vi "Background Color Read.vi"(8 "error in (no error)":errorcluster, 11 "3D Plot.lvclass in":refnum<class "3D Plot.lvclass">) -> (0 "error out":errorcluster, 1 "Plot Area Color":u32(colorbox), 3 "3D Plot.lvclass out":refnum<class "3D Plot.lvclass">)   [LabVIEW 2020, in "3D Plot.lvclass"]
uses:
  <vilib>/Math Plots/3D Math Plots/3D Plot/3D Plot/3D Plot.lvclass
  <vilib>/Math Plots/3D Math Plots/3D Plot/3D Plot/3D Plot.lvclass/3D Plot.ctl
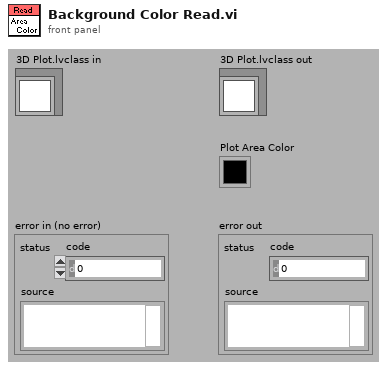
[diagram p1: front panel]
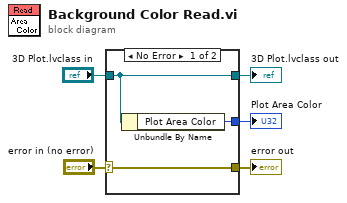
[diagram p0: block diagram]
diagram:
  n1 = case shown="No Error" "error in (no error)" {
    selector: "error in (no error)" -> [w7 w9]
    tunnel: [w8 _] -> w5
    tunnel: "3D Plot.lvclass in" -> [w6 w10]
    tunnel: [w7 w9] -> w2
    tunnel: [w6 w10] -> w1
    frame No Error {
      n2 = Unbundle By Name(w6) -> ("Plot Area Color"=w8:u32)
    }
    frame Error {
    }
  }
  "error out" <- w2
  "Plot Area Color" <- w5
  "3D Plot.lvclass out" <- w1
